vi "Result_Test.vi"(8 "error in (no error)":errorcluster caption="entrée d'erreur (pas d'erreur)", 11 "Get_Voltage en entrée":refnum<class "P2056_Get_FW.lvclass">) -> (0 "error out":errorcluster caption="sortie d'erreur", 3 "Get_Voltage en sortie":refnum<class "P2056_Get_FW.lvclass">)   [LabVIEW 2020, in "Library Test.lvlib" / "P2056_Get_FW.lvclass"]
uses:
  P2056_Get_FW.lvclass
  C:/Users/ngarcin/OneDrive - Altyor/Standard TB/Class/Test/Test (Default)/Test (Default).lvclass
  JSON API/JSON Value/Set from JSON string.vi
  JSON API/JSON Value/JSON Value.lvclass
  P2056_Send_Command_UART.lvclass
  P2056_Get_FW.lvclass/P2056_Get_FW.ctl
  JSON API/Variant JSON/Variant JSON.lvlib
  JSON API/Get Polymorphic/JSON GetSet.lvlib
  Commun VI/Library Commun.lvlib
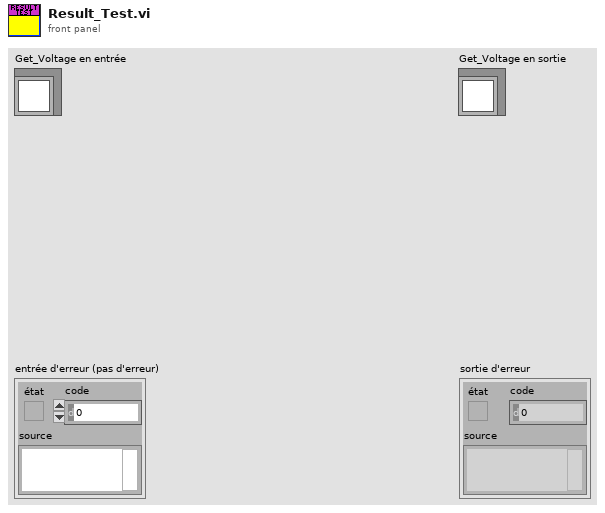
[diagram p1: front panel]
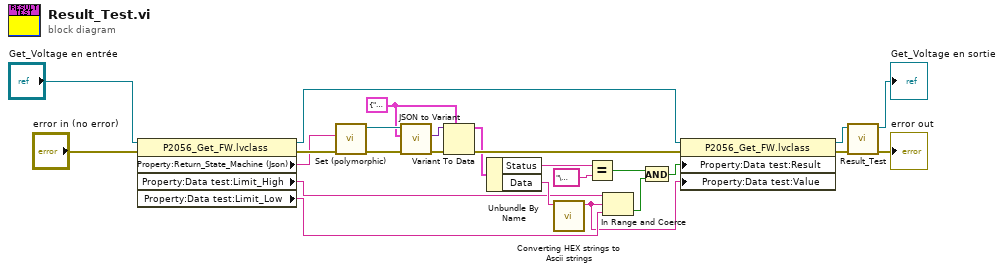
[diagram p0: block diagram]
diagram:
  w18 = cluster{"Data":string, "Status":string} {"Data"="", "Status"=""}
  n1 = property class="P2056_Get_FW.lvclass"(reference="Get_Voltage en entrée", error in="error in (no error)") -> (reference out=w23:refnum<class "P2056_Get_FW.lvclass">, error out=w17:errorcluster, "Property:Return_State_Machine (Json)"=w15:string, "Property:Data test:Limit_High"=w5:string, "Property:Data test:Limit_Low"=w4:string)
  n2 = call-poly "Set (polymorphic).vi"("error in (no error)"=w17, "JSON stream"=w15) -> ("error out"=w20:errorcluster, "JSON Value out"=w22:refnum<class "JSON Value.lvclass">)  [unwired: 7 in, 1 out]
  n3 = call "JSON to Variant.vi"("error in (no error)"=w20, "Variant (Data Type)"=w18, "JSON Value"=w22) -> ("error out"=w21:errorcluster, "Variant out"=w19:variant)  [unwired: 7 in]
  n4 = Variant To Data(error in=w21, type=w18, Variant=w19) -> (data=w14:cluster{"Data":string, "Status":string}, error out=w16:errorcluster)
  n5 = Unbundle By Name(w14) -> ("Status"=w13:string, "Data"=w6:string)
  n6 = call "Converting HEX strings to Ascii strings.vi"("chaîne IN"=w6) -> ("Chaîne OUT"=w1:string)  [unwired: 9 in, 1 out]
  n7 = Equal?(x=w13, y="\u0000") -> (x = y?=w11:bool)
  n8 = In Range and Coerce(upper limit=w5, x=w1, lower limit=w4) -> (In Range?=w2:bool)  [unwired: 1 out]
  n9 = And(x=w11, y=w2) -> (x .and. y?=w3:bool)
  n10 = property class="P2056_Get_FW.lvclass"(reference=w23, error in=w16, "Property:Data test:Result"=w3, "Property:Data test:Value"=w1) -> (reference out=w10:refnum<class "P2056_Get_FW.lvclass">, error out=w9:errorcluster)
  n11 = call-parent "Result_Test.vi"("error in (no error)"=w9, "Get_Voltage en entrée"=w10) -> ("error out"=→"error out":errorcluster, "Get_Voltage en sortie"=→"Get_Voltage en sortie":refnum<class "P2056_Get_FW.lvclass">)  [unwired: 8 in]
